vi "JSON Context Check.vi"(10 "Invalid in":bool, 11 "Parse Tokens in":T1[](array[typedef])) -> (2 "Invalid out":bool, 3 "tokens":cluster{"token type":T3, T1}[](array[cluster]))   [LabVIEW 2020, in "Multi Error Cluster.lvlib"]
doc: "Apply JSON context rules to the input tokens."
uses:
  <vilib>/MultiError/TokenizeJSON/Multi Error Cluster.lvlib
  <vilib>/MultiError/TokenizeJSON/JSON Token Values.ctl
  <vilib>/MultiError/Errors Cluster Multiple Errors/JSON Token Descriptor.ctl
  <vilib>/MultiError/TokenizeJSON/JSON Raw Token Values.ctl
  <vilib>/MultiError/TokenizeJSON/JSON Token Identifier.ctl
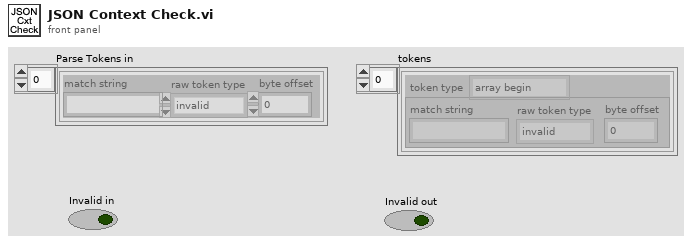
[diagram p1: front panel]
types:
  T1 = typedef "Multi Error Cluster.lvlib/JSON Token Descriptor.ctl" = cluster{"match string":string, "raw token type":T2, "byte offset ":i32}
  T2 = typedef "Multi Error Cluster.lvlib/JSON Raw Token Values.ctl" = enum32{"{", "}", "[", "]", ",", ":", "\"", "number", "string", "true", "false", "null", "invalid"}
  T3 = typedef "Multi Error Cluster.lvlib/JSON Token Values.ctl" = enum32{"array begin", "array end", "object begin", "object end", "value", "invalid", "name"}
  T4 = typedef "Multi Error Cluster.lvlib/JSON Token Identifier.ctl" = enum16{"Value Begin", "Value Complete", "Object Begin", "Object First", "Object String", "Object Value", "Object Complete", "Array Value", "Array First Value", "Array Complete", "Invalid"}
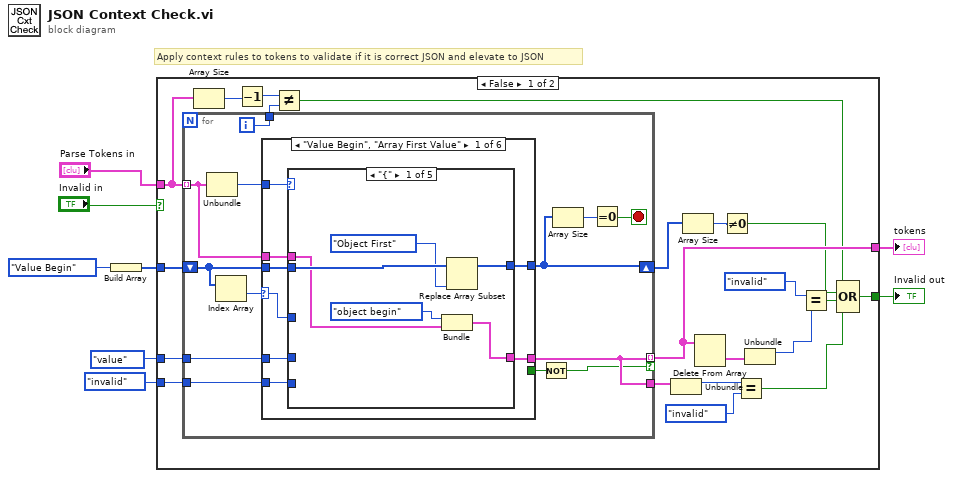
[diagram p0: block diagram]
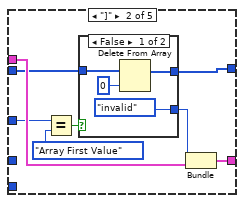
[diagram p2: hidden frame]
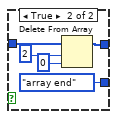
[diagram p3: hidden frame]
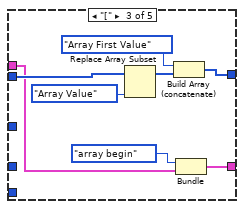
[diagram p4: hidden frame]
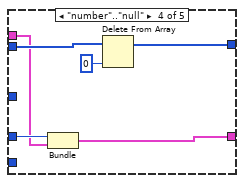
[diagram p5: hidden frame]
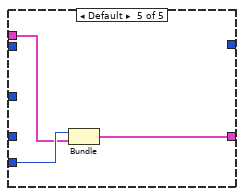
[diagram p6: hidden frame]
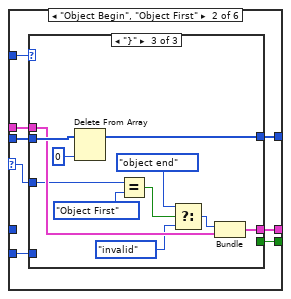
[diagram p7: hidden frame]
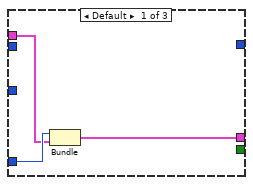
[diagram p8: hidden frame]
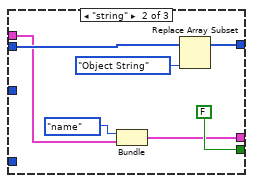
[diagram p9: hidden frame]
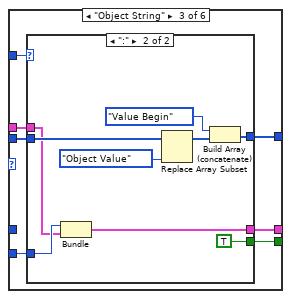
[diagram p10: hidden frame]
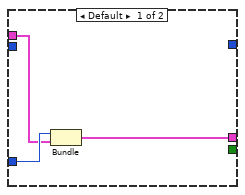
[diagram p11: hidden frame]
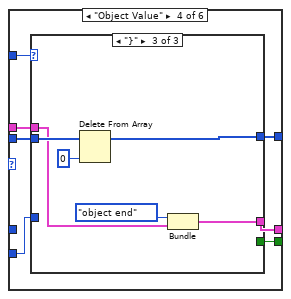
[diagram p12: hidden frame]
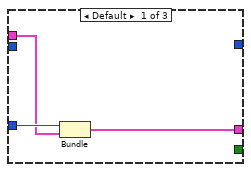
[diagram p13: hidden frame]
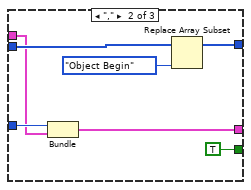
[diagram p14: hidden frame]
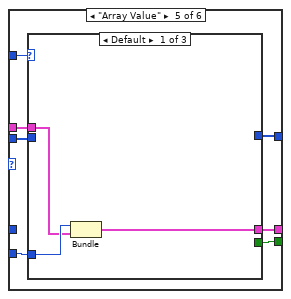
[diagram p15: hidden frame]
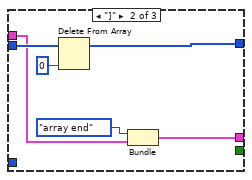
[diagram p16: hidden frame]
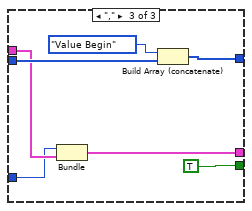
[diagram p17: hidden frame]
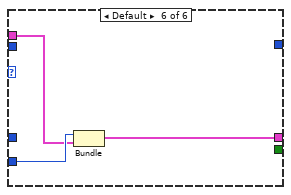
[diagram p18: hidden frame]
diagram:
  # "Apply context rules to tokens to validate if it is correct JSON and elevate to JSON"
  n1 = Build Array(JSON_Token_Identifier."Value Begin") -> (w2:T4[])
  n2 = case shown="False" "Invalid in" {
    selector: "Invalid in" -> [_ w188]
    tunnel: "Parse Tokens in" -> [w13 _]
    tunnel: w2 -> [w29 _]
    tunnel: JSON_Token_Values."value" ("token type") -> [w28 _]
    tunnel: JSON_Token_Values."invalid" ("token type") -> [w27 _]
    tunnel: [w26 _] -> w3
    tunnel: [w23 w188] -> w8
    frame False {
      n3 = for {
        tunnel: w13 -> [w32] mode=indexing
        shift-right: [w40] -> w22
        shift-left: w29 -> [w41]
        tunnel: [w35] -> w26 mode=indexing if=w33
        tunnel: w28 -> [w37]
        tunnel: w27 -> [w36]
        tunnel: [w35] -> w17
        tunnel: [w31] -> w10
        i -> [w31]
        stop <- w38 stop-if-true
        n4 = Unbundle(w32) -> ("raw token type"=w42:T2)  [unwired: 2 out]
        n5 = Index Array(array=w41) -> (element=w30:T4)  [unwired: 1 in]
        n6 = case shown="\"Value Begin\", \"Array First Value\"" w30 {
          selector: w30 -> [w43 w91 _ _ _ _]
          tunnel: w42 -> [w50 w98 w126 w145 w168 _]
          tunnel: [w49 w97 w125 w144 w166 _] -> w40
          tunnel: [w48 w96 w124 w143 w165 w187] -> w35
          tunnel: w41 -> [w47 w95 w123 w142 w167 _]
          tunnel: w37 -> [w46 _ _ _ _ _]
          tunnel: w36 -> [w45 w94 w122 w141 w164 w186]
          tunnel: [_ w93 w121 w140 w163 _] -> w34
          tunnel: w32 -> [w44 w92 w120 w139 w162 w185]
          frame "Value Begin", "Array First Value" {
            n7 = case shown="\"{\"" w50 {
              tunnel: [w55 w61 w79 w87 _] -> w49
              tunnel: [w52 w63 w77 w83 w89] -> w48
              tunnel: w46 -> [_ _ _ w84 _]
              tunnel: w47 -> [w56 w62 w81 w86 _]
              tunnel: w45 -> [_ _ _ _ w90]
              tunnel: w44 -> [w53 w64 w76 w82 w88]
              tunnel: w43 -> [_ w60 _ _ _]
              frame "{" {
                n8 = Bundle("token type"=JSON_Token_Values."object begin", w53) -> (w52:cluster{"token type":T3, T1})  [unwired: 1 in]
                n9 = Replace Array Subset(array=w56, new element=JSON_Token_Identifier."Object First") -> (w55:T4[])  [unwired: 1 in]
              }
              frame "]" {
                n10 = Equal?(x=w60, y=JSON_Token_Identifier."Array First Value") -> (x = y?=w58:bool)
                n11 = case shown="False" w58 {
                  tunnel: w62 -> [w66 w73]
                  tunnel: [w65 w72] -> w61
                  tunnel: [JSON_Token_Values."invalid" ("token type") JSON_Token_Values."array end" ("token type")] -> w57
                  frame False {
                    n12 = Delete From Array(array=w66, index=0) -> (array with subset deleted=w65:T4[])  [unwired: 1 in, 1 out]
                  }
                  frame True {
                    n13 = Delete From Array(array=w73, length=2 ("index"), index=0) -> (array with subset deleted=w72:T4[])  [unwired: 1 out]
                  }
                }
                n14 = Bundle("token type"=w57, w64) -> (w63:cluster{"token type":T3, T1})  [unwired: 1 in]
              }
              frame "[" {
                n15 = Replace Array Subset(array=w81, new element=JSON_Token_Identifier."Array Value") -> (w80:T4[])  [unwired: 1 in]
                n16 = Build Array (concatenate)(JSON_Token_Identifier."Array First Value", w80) -> (w79:T4[])
                n17 = Bundle("token type"=JSON_Token_Values."array begin", w76) -> (w77:cluster{"token type":T3, T1})  [unwired: 1 in]
              }
              frame "number".."null" {
                n18 = Bundle("token type"=w84, w82) -> (w83:cluster{"token type":T3, T1})  [unwired: 1 in]
                n19 = Delete From Array(array=w86, index=0) -> (array with subset deleted=w87:T4[])  [unwired: 1 in, 1 out]
              }
              frame Default {
                n20 = Bundle("token type"=w90, w88) -> (w89:cluster{"token type":T3, T1})  [unwired: 1 in]
              }
            }
          }
          frame "Object Begin", "Object First" {
            n21 = case shown="\"}\"" w98 {
              tunnel: [_ w107 w118] -> w97
              tunnel: [w100 w105 w116] -> w96
              tunnel: w95 -> [_ w108 w119]
              tunnel: w94 -> [w101 _ _]
              tunnel: [_ FALSE _] -> w93
              tunnel: w92 -> [w99 w104 w115]
              tunnel: w91 -> [_ _ w109]
              frame Default {
                n22 = Bundle("token type"=w101, w99) -> (w100:cluster{"token type":T3, T1})  [unwired: 1 in]
              }
              frame "string" {
                n23 = Bundle("token type"=JSON_Token_Values."name", w104) -> (w105:cluster{"token type":T3, T1})  [unwired: 1 in]
                n24 = Replace Array Subset(array=w108, new element=JSON_Token_Identifier."Object String") -> (w107:T4[])  [unwired: 1 in]
              }
              frame "}" {
                n25 = Delete From Array(array=w119, index=0) -> (array with subset deleted=w118:T4[])  [unwired: 1 in, 1 out]
                n26 = Equal?(x=w109, y=JSON_Token_Identifier."Object First") -> (x = y?=w113:bool)
                n27 = Select(t=JSON_Token_Values."object end" ("token type"), s=w113, f=JSON_Token_Values."invalid" ("token type")) -> (s? t:f=w111:T3)
                n28 = Bundle("token type"=w111, w115) -> (w116:cluster{"token type":T3, T1})  [unwired: 1 in]
              }
            }
          }
          frame "Object String" {
            n29 = case shown="\":\"" w126 {
              tunnel: [_ w136] -> w125
              tunnel: [w129 w134] -> w124
              tunnel: w123 -> [_ w138]
              tunnel: w122 -> [w128 w133]
              tunnel: [_ TRUE] -> w121
              tunnel: w120 -> [w127 w132]
              frame Default {
                n30 = Bundle("token type"=w128, w127) -> (w129:cluster{"token type":T3, T1})  [unwired: 1 in]
              }
              frame ":" {
                n31 = Bundle("token type"=w133, w132) -> (w134:cluster{"token type":T3, T1})  [unwired: 1 in]
                n32 = Replace Array Subset(array=w138, new element=JSON_Token_Identifier."Object Value") -> (w137:T4[])  [unwired: 1 in]
                n33 = Build Array (concatenate)(JSON_Token_Identifier."Value Begin", w137) -> (w136:T4[])
              }
            }
          }
          frame "Object Value" {
            n34 = case shown="\"}\"" w145 {
              tunnel: [_ w154 w161] -> w144
              tunnel: [w148 w151 w158] -> w143
              tunnel: w142 -> [_ w155 w160]
              tunnel: w141 -> [w147 w152 _]
              tunnel: [_ TRUE _] -> w140
              tunnel: w139 -> [w146 w150 w156]
              frame Default {
                n35 = Bundle("token type"=w147, w146) -> (w148:cluster{"token type":T3, T1})  [unwired: 1 in]
              }
              frame "," {
                n36 = Bundle("token type"=w152, w150) -> (w151:cluster{"token type":T3, T1})  [unwired: 1 in]
                n37 = Replace Array Subset(array=w155, new element=JSON_Token_Identifier."Object Begin") -> (w154:T4[])  [unwired: 1 in]
              }
              frame "}" {
                n38 = Delete From Array(array=w160, index=0) -> (array with subset deleted=w161:T4[])  [unwired: 1 in, 1 out]
                n39 = Bundle("token type"=JSON_Token_Values."object end", w156) -> (w158:cluster{"token type":T3, T1})  [unwired: 1 in]
              }
            }
          }
          frame "Array Value" {
            n40 = case shown="Default" w168 {
              tunnel: [_ w176 w183] -> w166
              tunnel: [w171 w174 w181] -> w165
              tunnel: w167 -> [_ w177 w184]
              tunnel: w164 -> [w170 _ w179]
              tunnel: [_ _ TRUE] -> w163
              tunnel: w162 -> [w169 w172 w180]
              frame Default {
                n41 = Bundle("token type"=w170, w169) -> (w171:cluster{"token type":T3, T1})  [unwired: 1 in]
              }
              frame "]" {
                n42 = Delete From Array(array=w177, index=0) -> (array with subset deleted=w176:T4[])  [unwired: 1 in, 1 out]
                n43 = Bundle("token type"=JSON_Token_Values."array end", w172) -> (w174:cluster{"token type":T3, T1})  [unwired: 1 in]
              }
              frame "," {
                n44 = Bundle("token type"=w179, w180) -> (w181:cluster{"token type":T3, T1})  [unwired: 1 in]
                n45 = Build Array (concatenate)(JSON_Token_Identifier."Value Begin", w184) -> (w183:T4[])
              }
            }
          }
          frame Default {
            n46 = Bundle("token type"=w186, w185) -> (w187:cluster{"token type":T3, T1})  [unwired: 1 in]
          }
        }
        n47 = Not(x=w34) -> (.not. x?=w33:bool)
        n48 = Array Size(array=w40) -> (size(s)=w39:i32)
        n49 = Equal To 0?(x=w39) -> (x = 0?=w38:bool)
      }
      n50 = Array Size(array=w13) -> (size(s)=w12:i32)
      n51 = Decrement(x=w12) -> (x-1=w11:i32)
      n52 = Not Equal?(x=w11, y=w10) -> (x != y?=w9:bool)
      n53 = Unbundle(w17) -> ("token type"=w16:T3)  [unwired: 1 out]
      n54 = Array Size(array=w22) -> (size(s)=w21:i32)
      n55 = Delete From Array(array=w26) -> (deleted portion=w15:cluster{"token type":T3, T1})  [unwired: 2 in, 1 out]
      n56 = Not Equal To 0?(x=w21) -> (x != 0?=w20:bool)
      n57 = Equal?(x=w16, y=JSON_Token_Values."invalid" ("token type")) -> (x = y?=w18:bool)
      n58 = Unbundle(w15) -> ("token type"=w14:T3)  [unwired: 1 out]
      n59 = Equal?(x=JSON_Token_Values."invalid" ("token type"), y=w14) -> (x = y?=w24:bool)
      n60 = Compound Arithmetic op=OR(w9, w20, w24, w18) -> (w23:bool)
    }
    frame True {
    }
  }
  "Invalid out" <- w8
  "tokens" <- w3
